vi "TriggerDialog.vi"(8 "Error In":errorcluster, 11 "Trigger Configuration In":T4={"Arm"={"Source"=enum."Hold", "Count"=1, "Infinite?"=FALSE}, "Scan"={"Source"=enum."Hold", "Count"=1, "Infinite?"=FALSE, "Delay (sec)"=0.0, "Interval (sec)"=0.0}, "Channel"={"Source"=enum."Hold", "Count"=1, "Infinite?"=FALSE, "Auto Count?"=FALSE, "Delay (sec)"=0.0, "Interval (sec)"=0.0}} {"Arm"."Count" min=1 max=99999 step=1}) -> (0 "Error Out":errorcluster, 2 "Cancelled?":bool, 3 "Trigger Configuration Out":T4={"Arm"={"Source"=enum."Hold", "Count"=1, "Infinite?"=FALSE}, "Scan"={"Source"=enum."Hold", "Count"=0, "Infinite?"=FALSE, "Delay (sec)"=0.0, "Interval (sec)"=0.0}, "Channel"={"Source"=enum."Hold", "Count"=0, "Infinite?"=FALSE, "Auto Count?"=FALSE, "Delay (sec)"=0.0, "Interval (sec)"=0.0}} {"Arm"."Count" min=1 max=99999 step=1})   [LabVIEW 2012]
uses:
  TriggerConfiguration.ctl
  TriggerArmConfiguration.ctl
  driver/Public/Controls/ArmSource.ctl
  TriggerScanConfiguration.ctl
  driver/Public/Controls/ScanSource.ctl
  TriggerChannelConfiguration.ctl
  driver/Public/Controls/TriggerSource.ctl
  libs/LV-Utilities/LV-Utilities.lvlib
  driver/Keithley-7001.lvlib
panel:
  in  "Channel Interval (sec)":dbl format="%_4p"
  in  "Channel Delay (sec)":dbl format="%_4p"
  in  "Channel Count":u32=1 min=1 max=9999 step=1
  in  "Channel Count Limit":enum16{"Auto", "Finite", "Infinite"}(ring)
  in  "Channel Source":T1(ring)
  in  "Scan Interval (sec)":dbl format="%_4p"
  in  "Scan Delay (sec)":dbl format="%_4p"
  in  "Scan Count":u32=1 min=1 max=9999 step=1
  in  "Scan Count Limit":enum16{"Finite", "Infinite"}(ring)
  in  "Scan Source":T2(ring)
  in  "Arm Count":u32=1 min=1 max=9999 step=1
  in  "Arm Count Limit":enum16{"Finite", "Infinite"}(ring)
  in  "Arm Source":T3(ring)
  in  "CANCEL":bool
  in  "DONE":bool
  # "CHANNEL"
  # "Interval"
  # "Delay"
  # "Count"
  # "Count Limit"
  # "Source"
  # "SCAN"
  # "Interval"
  # "Delay"
  # "Count"
  # "Count Limit"
  # "Source"
  # "ARM"
  # "Count"
  # "Count Limit"
  # "Source"
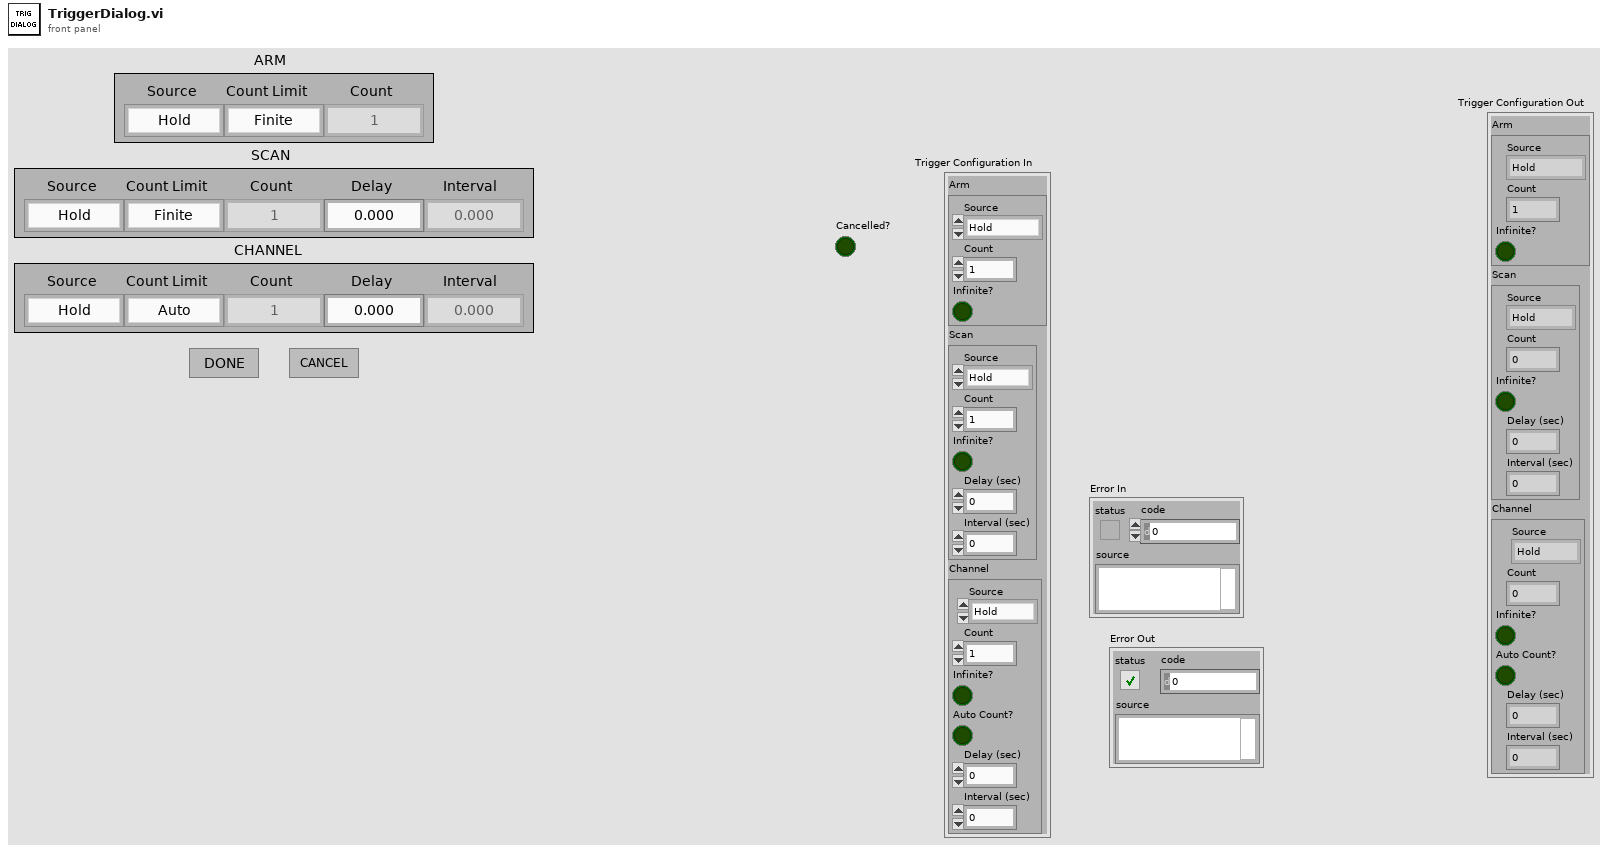
[diagram p1: front panel]
types:
  T1 = enum16{"Hold", "Imm.", "Manual", "Bus", "TLink", "External", "Timer"}
  T2 = enum16{"Hold", "Imm.", "Timer", "Manual", "Bus", "TLink", "External"}
  T3 = enum16{"Hold", "Imm.", "Manual", "Bus", "TLink", "External"}
  T4 = typedef "TriggerConfiguration.ctl" = cluster{"Arm":T5, "Scan":T7, "Channel":T9}
  T5 = typedef "TriggerArmConfiguration.ctl" = cluster{"Source":T6, "Count":u32, "Infinite?":bool}
  T6 = typedef "Keithley-7001.lvlib/ArmSource.ctl" = enum16{"Hold", "Immediate", "Manual", "Bus", "TLink", "External"}
  T7 = typedef "TriggerScanConfiguration.ctl" = cluster{"Source":T8, "Count":u32, "Infinite?":bool, "Delay (sec)":dbl, "Interval (sec)":dbl}
  T8 = typedef "Keithley-7001.lvlib/ScanSource.ctl" = enum16{"Hold", "Immediate", "Timer", "Manual", "Bus", "TLink", "External"}
  T9 = typedef "TriggerChannelConfiguration.ctl" = cluster{"Source":T10, "Count":u32, "Infinite?":bool, "Auto Count?":bool, "Delay (sec)":dbl, "Interval (sec)":dbl}
  T10 = typedef "Keithley-7001.lvlib/TriggerSource.ctl" = enum16{"Hold", "Immediate", "Manual", "Bus", "TLink", "External", "Timer"}
  T11 = enum8{"Enabled", "Disabled", "Disabled and Grayed Out"}
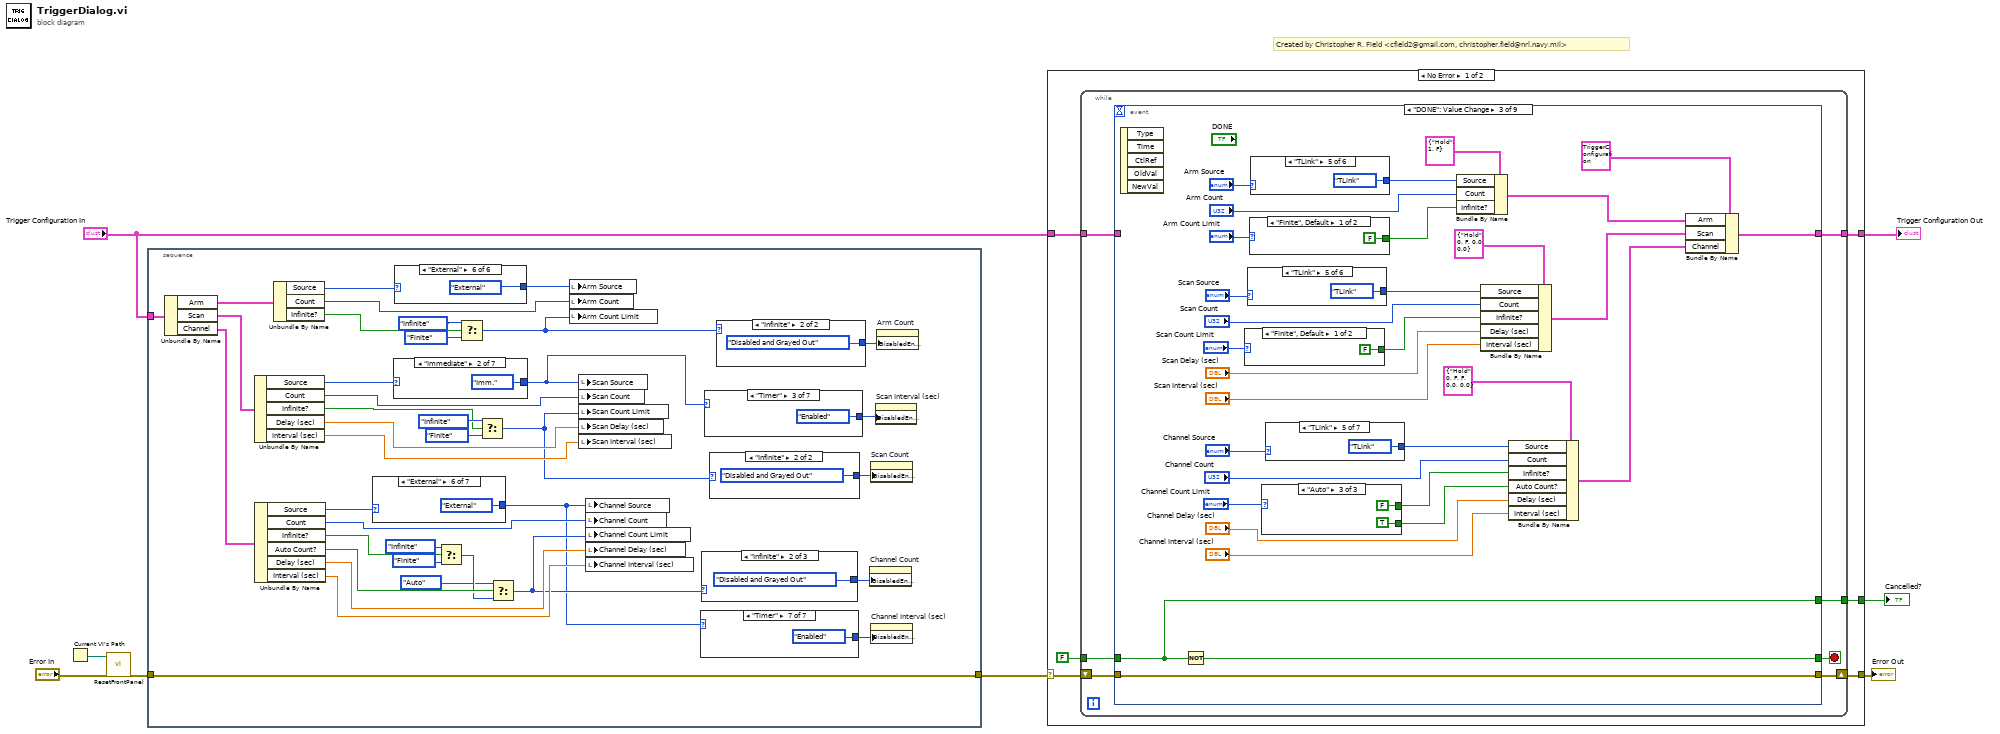
[diagram p0: block diagram]
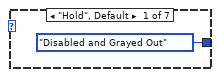
[diagram p2: hidden frame]
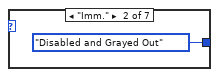
[diagram p3: hidden frame]
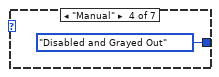
[diagram p4: hidden frame]
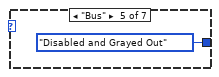
[diagram p5: hidden frame]
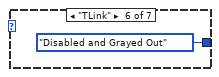
[diagram p6: hidden frame]
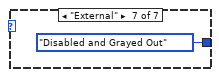
[diagram p7: hidden frame]
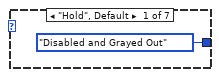
[diagram p8: hidden frame]
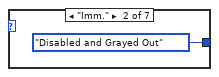
[diagram p9: hidden frame]
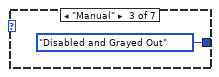
[diagram p10: hidden frame]
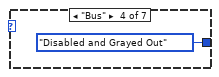
[diagram p11: hidden frame]
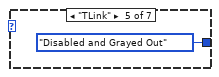
[diagram p12: hidden frame]
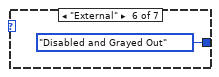
[diagram p13: hidden frame]
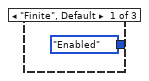
[diagram p14: hidden frame]
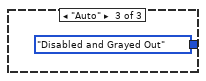
[diagram p15: hidden frame]
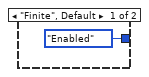
[diagram p16: hidden frame]
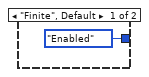
[diagram p17: hidden frame]
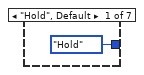
[diagram p18: hidden frame]
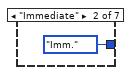
[diagram p19: hidden frame]
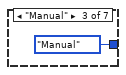
[diagram p20: hidden frame]
diagram:
  # "Created by Christopher R. Field <cfield2@gmail.com, christopher.field@nrl.navy.mil>"
  n1 = Current VI's Path() -> (path=w8:path)
  n2 = call "ResetFrontPanel.vi"("Error In"="Error In", "VI Path"=w8) -> ("Error Out"=w6:errorcluster)  [unwired: 9 in]
  n3 = stacked-sequence {
    tunnel: w6 -> [w46]
    tunnel: [w46] -> w5
    tunnel: "Trigger Configuration In" -> [w45]
    frame #0 {
      n4 = Unbundle By Name(w45) -> ("Arm"=w44:T5, "Scan"=w43:T7, "Channel"=w42:T9)
      n5 = Unbundle By Name(w43) -> ("Source"=w36:T8, "Count"=w35:u32, "Infinite?"=w32:bool, "Delay (sec)"=w31:dbl, "Interval (sec)"=w30:dbl)
      n6 = Unbundle By Name(w42) -> ("Source"=w29:T10, "Count"=w28:u32, "Infinite?"=w27:bool, "Auto Count?"=w26:bool, "Delay (sec)"=w21:dbl, "Interval (sec)"=w20:dbl)
      n7 = Unbundle By Name(w44) -> ("Source"=w41:T6, "Count"=w40:u32, "Infinite?"=w39:bool)
      n8 = case shown="\"External\"" w29 {
        tunnel: [T1."Hold" ("Channel Source") T1."Imm." ("Channel Source") T1."Manual" ("Channel Source") T1."Bus" ("Channel Source") T1."TLink" ("Channel Source") T1."External" ("Channel Source") T1."Timer" ("Channel Source")] -> w12
        frame "Hold", Default {
        }
        frame "Immediate" {
        }
        frame "Manual" {
        }
        frame "Bus" {
        }
        frame "TLink" {
        }
        frame "External" {
        }
        frame "Timer" {
        }
      }
      n9 = case shown="\"Immediate\"" w36 {
        tunnel: [T2."Hold" ("Scan Source") T2."Imm." ("Scan Source") T2."Timer" ("Scan Source") T2."Manual" ("Scan Source") T2."Bus" ("Scan Source") T2."TLink" ("Scan Source") T2."External" ("Scan Source")] -> w10
        frame "Hold", Default {
        }
        frame "Immediate" {
        }
        frame "Timer" {
        }
        frame "Manual" {
        }
        frame "Bus" {
        }
        frame "TLink" {
        }
        frame "External" {
        }
      }
      n10 = case shown="\"External\"" w41 {
        tunnel: [T3."Hold" ("Arm Source") T3."Imm." ("Arm Source") T3."Manual" ("Arm Source") T3."Bus" ("Arm Source") T3."TLink" ("Arm Source") T3."External" ("Arm Source")] -> w19
        frame "Hold", Default {
        }
        frame "Immediate" {
        }
        frame "Manual" {
        }
        frame "Bus" {
        }
        frame "TLink" {
        }
        frame "External" {
        }
      }
      n11 = Select(t=enum16{"Auto", "Finite", "Infinite"}."Infinite" ("Channel Count Limit"), s=w27, f=enum16{"Auto", "Finite", "Infinite"}."Finite" ("Channel Count Limit")) -> (s? t:f=w25:enum16{"Auto", "Finite", "Infinite"})
      n12 = Select(t=enum16{"Finite", "Infinite"}."Infinite" ("Arm Count Limit"), s=w39, f=enum16{"Finite", "Infinite"}."Finite") -> (s? t:f=w18:enum16{"Finite", "Infinite"})
      n13 = Select(t=enum16{"Finite", "Infinite"}."Infinite" ("Arm Count Limit"), s=w32, f=enum16{"Finite", "Infinite"}."Finite") -> (s? t:f=w15:enum16{"Finite", "Infinite"})
      n14 = Select(t=enum16{"Auto", "Finite", "Infinite"}."Auto" ("Channel Count Limit"), s=w26, f=w25) -> (s? t:f=w13:enum16{"Auto", "Finite", "Infinite"})
      n15 = local write "Arm Source"(w19) -> ()
      n16 = local write "Arm Count"(w40) -> ()
      n17 = local write "Arm Count Limit"(w18) -> ()
      n18 = local write "Scan Source"(w10) -> ()
      n19 = local write "Scan Count"(w35) -> ()
      n20 = local write "Scan Count Limit"(w15) -> ()
      n21 = local write "Scan Delay (sec)"(w31) -> ()
      n22 = local write "Scan Interval (sec)"(w30) -> ()
      n23 = local write "Channel Source"(w12) -> ()
      n24 = local write "Channel Count"(w28) -> ()
      n25 = local write "Channel Count Limit"(w13) -> ()
      n26 = local write "Channel Delay (sec)"(w21) -> ()
      n27 = local write "Channel Interval (sec)"(w20) -> ()
      n28 = case shown="\"Timer\"" w12 {
        tunnel: [T11."Disabled and Grayed Out" ("Disabled") T11."Disabled and Grayed Out" ("Disabled") T11."Disabled and Grayed Out" ("Disabled") T11."Disabled and Grayed Out" ("Disabled") T11."Disabled and Grayed Out" ("Disabled") T11."Disabled and Grayed Out" ("Disabled") T11."Enabled" ("Disabled")] -> w11
        frame "Hold", Default {
        }
        frame "Imm." {
        }
        frame "Manual" {
        }
        frame "Bus" {
        }
        frame "TLink" {
        }
        frame "External" {
        }
        frame "Timer" {
        }
      }
      n29 = case shown="\"Infinite\"" w13 {
        tunnel: [T11."Enabled" ("Disabled") T11."Disabled and Grayed Out" ("Disabled") T11."Disabled and Grayed Out" ("Disabled")] -> w14
        frame "Finite", Default {
        }
        frame "Infinite" {
        }
        frame "Auto" {
        }
      }
      n30 = case shown="\"Timer\"" w10 {
        tunnel: [T11."Disabled and Grayed Out" ("Disabled") T11."Disabled and Grayed Out" ("Disabled") T11."Enabled" ("Disabled") T11."Disabled and Grayed Out" ("Disabled") T11."Disabled and Grayed Out" ("Disabled") T11."Disabled and Grayed Out" ("Disabled") T11."Disabled and Grayed Out" ("Disabled")] -> w9
        frame "Hold", Default {
        }
        frame "Imm." {
        }
        frame "Timer" {
        }
        frame "Manual" {
        }
        frame "Bus" {
        }
        frame "TLink" {
        }
        frame "External" {
        }
      }
      n31 = case shown="\"Infinite\"" w15 {
        tunnel: [T11."Enabled" ("Disabled") T11."Disabled and Grayed Out" ("Disabled")] -> w16
        frame "Finite", Default {
        }
        frame "Infinite" {
        }
      }
      n32 = case shown="\"Infinite\"" w18 {
        tunnel: [T11."Enabled" ("Disabled") T11."Disabled and Grayed Out" ("Disabled")] -> w17
        frame "Finite", Default {
        }
        frame "Infinite" {
        }
      }
      n33 = property on="Channel Count" class="DigNum (strict)"("DisabledEnum"=w14) -> ()  [unwired: 2 in, 2 out]
      n34 = property on="Scan Count" class="DigNum (strict)"("DisabledEnum"=w16) -> ()  [unwired: 2 in, 2 out]
      n35 = property on="Channel Interval (sec)" class="DigNum (strict)"("DisabledEnum"=w11) -> ()  [unwired: 2 in, 2 out]
      n36 = property on="Scan Interval (sec)" class="DigNum (strict)"("DisabledEnum"=w9) -> ()  [unwired: 2 in, 2 out]
      n37 = property on="Arm Count" class="DigNum (strict)"("DisabledEnum"=w17) -> ()  [unwired: 2 in, 2 out]
    }
  }
  n38 = case shown="No Error" w5 {
    selector: w5 -> [w93 w220]
    tunnel: [w92 w220] -> w4
    tunnel: "Trigger Configuration In" -> [w90 w219]
    tunnel: [w89 w219] -> w2
    tunnel: [w88 FALSE] -> w1
    frame No Error {
      n39 = while {
        shift-right: [w99] -> w92
        shift-left: w93 -> [w100]
        tunnel: FALSE -> [w98]
        tunnel: w90 -> [w96]
        tunnel: [w95] -> w89
        tunnel: [w94] -> w88
        stop <- w97 stop-if-true
        n40 = event shown="[2] \"DONE\": Value Change" {
          selector: _ -> [_ _ _ _ _ _ _ _ _]
          dyn-events: _ -> [_ _ _ _ _ _ _ _ _]
          timeout: _ -> [_ _ _ _ _ _ _ _ _]
          tunnel: w100 -> [w103 w107 w137 w171 w175 w183 w190 w203 w216]
          tunnel: [w103 w107 w137 w171 w175 w183 w190 w203 w216] -> w99
          tunnel: w98 -> [w101 w106 w136 w170 w176 w182 w192 w202 w215]
          tunnel: [w101 w104 w138 w170 w176 w182 w192 w202 w214] -> w97
          tunnel: w96 -> [w102 w105 _ w172 w177 w184 w191 w204 w217]
          tunnel: [w102 w105 w127 w172 w177 w184 w191 w204 w217] -> w95
          tunnel: [w101 w104 w136 w170 w176 w182 w192 w202 w214] -> w94
          event Timeout {
            n41 = event-data() -> ()  [unwired: 1 in, 2 out]
          }
          event Panel Close? {
            n42 = event-data() -> ()  [unwired: 1 in, 3 out]
            n43 = Not(x=w106) -> (.not. x?=w104:bool)
            n44 = event-data("Discard?"=w104) -> ()  [unwired: 1 in, 1 out]
          }
          event "DONE": Value Change {
            n45 = event-data() -> ()  [unwired: 1 in, 5 out]
            n46 = Not(x=w136) -> (.not. x?=w138:bool)
            n47 = case shown="\"Finite\", Default" "Scan Count Limit" {
              tunnel: [FALSE TRUE] -> w122
              frame "Finite", Default {
              }
              frame "Infinite" {
              }
            }
            n48 = case shown="\"TLink\"" "Scan Source" {
              tunnel: [ScanSource."Hold" ("Source") ScanSource."Immediate" ("Source") ScanSource."Manual" ("Source") ScanSource."Bus" ("Source") ScanSource."TLink" ("Source") ScanSource."External" ("Source")] -> w108
              frame "Hold", Default {
              }
              frame "Imm." {
              }
              frame "Manual" {
              }
              frame "Bus" {
              }
              frame "TLink" {
              }
              frame "External" {
              }
            }
            n49 = case shown="\"Finite\", Default" "Arm Count Limit" {
              tunnel: [FALSE TRUE] -> w129
              frame "Finite", Default {
              }
              frame "Infinite" {
              }
            }
            n50 = case shown="\"TLink\"" "Arm Source" {
              tunnel: [ArmSource."Hold" ("Source") ArmSource."Immediate" ("Source") ArmSource."Manual" ("Source") ArmSource."Bus" ("Source") ArmSource."TLink" ("Source") ArmSource."External" ("Source")] -> w132
              frame "Hold", Default {
              }
              frame "Imm." {
              }
              frame "Manual" {
              }
              frame "Bus" {
              }
              frame "TLink" {
              }
              frame "External" {
              }
            }
            n51 = case shown="\"Auto\"" "Channel Count Limit" {
              tunnel: [FALSE TRUE FALSE] -> w113
              tunnel: [FALSE FALSE TRUE] -> w112
              frame "Finite", Default {
              }
              frame "Infinite" {
              }
              frame "Auto" {
              }
            }
            n52 = case shown="\"TLink\"" "Channel Source" {
              tunnel: [TriggerSource."Hold" ("Source") TriggerSource."Immediate" ("Source") TriggerSource."Manual" ("Source") TriggerSource."Bus" ("Source") TriggerSource."TLink" ("Source") TriggerSource."External" ("Source") TriggerSource."Timer" ("Source")] -> w117
              frame "Hold", Default {
              }
              frame "Imm." {
              }
              frame "Manual" {
              }
              frame "Bus" {
              }
              frame "TLink" {
              }
              frame "External" {
              }
              frame "Timer" {
              }
            }
            n53 = Bundle By Name(cluster=T5 {"Source"=enum."Hold", "Count"=1, "Infinite?"=FALSE} ("Trigger Arm Configuration"), "Source"=w132, "Count"="Arm Count", "Infinite?"=w129) -> (w128:T5)
            n54 = Bundle By Name(cluster=T7 {"Source"=enum."Hold", "Count"=0, "Infinite?"=FALSE, "Delay (sec)"=0.0, "Interval (sec)"=0.0} ("Trigger Scan Configuration"), "Source"=w108, "Count"="Scan Count", "Infinite?"=w122, "Delay (sec)"="Scan Delay (sec)", "Interval (sec)"="Scan Interval (sec)") -> (w119:T7)
            n55 = Bundle By Name(cluster=T9 {"Source"=enum."Hold", "Count"=0, "Infinite?"=FALSE, "Auto Count?"=FALSE, "Delay (sec)"=0.0, "Interval (sec)"=0.0} ("Trigger Channel Configuration"), "Source"=w117, "Count"="Channel Count", "Infinite?"=w113, "Auto Count?"=w112, "Delay (sec)"="Channel Delay (sec)", "Interval (sec)"="Channel Interval (sec)") -> (w109:T9)
            n56 = Bundle By Name(cluster=T4 {"Arm"={"Source"=enum."Hold", "Count"=1, "Infinite?"=FALSE}, "Scan"={"Source"=enum."Hold", "Count"=0, "Infinite?"=FALSE, "Delay (sec)"=0.0, "Interval (sec)"=0.0}, "Channel"={"Source"=enum."Hold", "Count"=0, "Infinite?"=FALSE, "Auto Count?"=FALSE, "Delay (sec)"=0.0, "Interval (sec)"=0.0}} ("Trigger Configuration"), "Arm"=w128, "Scan"=w119, "Channel"=w109) -> (w127:T4)
          }
          event "Arm Count Limit": Value Change {
            n57 = event-data() -> ("NewVal"=w169:enum16{"Finite", "Infinite"})  [unwired: 1 in, 4 out]
            n58 = case shown="\"Finite\", Default" w169 {
              tunnel: [T11."Enabled" ("Disabled") T11."Disabled and Grayed Out" ("Disabled")] -> w168
              frame "Finite", Default {
              }
              frame "Infinite" {
              }
            }
            n59 = property on="Arm Count" class="DigNum (strict)"("DisabledEnum"=w168) -> ()  [unwired: 2 in, 2 out]
          }
          event "Scan Count Limit": Value Change {
            n60 = event-data() -> ("NewVal"=w178:enum16{"Finite", "Infinite"})  [unwired: 1 in, 4 out]
            n61 = case shown="\"Finite\", Default" w178 {
              tunnel: [T11."Enabled" ("Disabled") T11."Disabled and Grayed Out" ("Disabled")] -> w179
              frame "Finite", Default {
              }
              frame "Infinite" {
              }
            }
            n62 = property on="Scan Count" class="DigNum (strict)"("DisabledEnum"=w179) -> ()  [unwired: 2 in, 2 out]
          }
          event "Channel Count Limit": Value Change {
            n63 = event-data() -> ("NewVal"=w185:enum16{"Auto", "Finite", "Infinite"})  [unwired: 1 in, 4 out]
            n64 = case shown="\"Auto\"" w185 {
              tunnel: [T11."Enabled" ("Disabled") T11."Disabled and Grayed Out" ("Disabled") T11."Disabled and Grayed Out" ("Disabled")] -> w186
              frame "Finite", Default {
              }
              frame "Infinite" {
              }
              frame "Auto" {
              }
            }
            n65 = property on="Channel Count" class="DigNum (strict)"("DisabledEnum"=w186) -> ()  [unwired: 2 in, 2 out]
          }
          event "Scan Source": Value Change {
            n66 = event-data() -> ("NewVal"=w193:T2)  [unwired: 1 in, 4 out]
            n67 = case shown="\"Timer\"" w193 {
              tunnel: [T11."Disabled and Grayed Out" ("Disabled") T11."Disabled and Grayed Out" ("Disabled") T11."Enabled" ("Disabled") T11."Disabled and Grayed Out" ("Disabled") T11."Disabled and Grayed Out" ("Disabled") T11."Disabled and Grayed Out" ("Disabled") T11."Disabled and Grayed Out" ("Disabled")] -> w194
              frame "Hold", Default {
              }
              frame "Imm." {
              }
              frame "Timer" {
              }
              frame "Manual" {
              }
              frame "Bus" {
              }
              frame "TLink" {
              }
              frame "External" {
              }
            }
            n68 = property on="Scan Interval (sec)" class="DigNum (strict)"("DisabledEnum"=w194) -> ()  [unwired: 2 in, 2 out]
          }
          event "Channel Source": Value Change {
            n69 = event-data() -> ("NewVal"=w205:T1)  [unwired: 1 in, 4 out]
            n70 = case shown="\"Timer\"" w205 {
              tunnel: [T11."Disabled and Grayed Out" ("Disabled") T11."Disabled and Grayed Out" ("Disabled") T11."Disabled and Grayed Out" ("Disabled") T11."Disabled and Grayed Out" ("Disabled") T11."Disabled and Grayed Out" ("Disabled") T11."Disabled and Grayed Out" ("Disabled") T11."Enabled" ("Disabled")] -> w206
              frame "Hold", Default {
              }
              frame "Imm." {
              }
              frame "Manual" {
              }
              frame "Bus" {
              }
              frame "TLink" {
              }
              frame "External" {
              }
              frame "Timer" {
              }
            }
            n71 = property on="Channel Interval (sec)" class="DigNum (strict)"("DisabledEnum"=w206) -> ()  [unwired: 2 in, 2 out]
          }
          event "CANCEL": Value Change {
            n72 = event-data() -> ()  [unwired: 1 in, 5 out]
            n73 = Not(x=w215) -> (.not. x?=w214:bool)
          }
        }
      }
    }
    frame Error {
    }
  }
  "Error Out" <- w4
  "Trigger Configuration Out" <- w2
  "Cancelled?" <- w1
